vi "Image Label.vi"() -> ()   [LabVIEW 2016]
doc: "This example shows how to label a binary image that contains multiple particles. The labeling process assigns a unique value to all the pixels that belong to a particle. Some processing functions in NI Vision require the input binary image to be labeled."
uses:
  <vilib>/vision/NI_Vision_Development_Module.lvlib
panel:
  out "Number of Particles Found":i32
  out "Extracted Image":T1(plugin-control) caption="Extracted Image (displayed using binary palette)"
  out "Image Source":T1(plugin-control)
  in  "Threshold Values":T2={"Minimum Value"=0.0, "Maximum Value"=150.0}
  in  "Connectivity":bool
  # "Overview: Demonstrates how to threshold an image, smooth the contours of the particles found using an Auto-Median morphological operator, and label the image.\nRequirements: NI Vision Development Module\nInstructions: Run the VI."
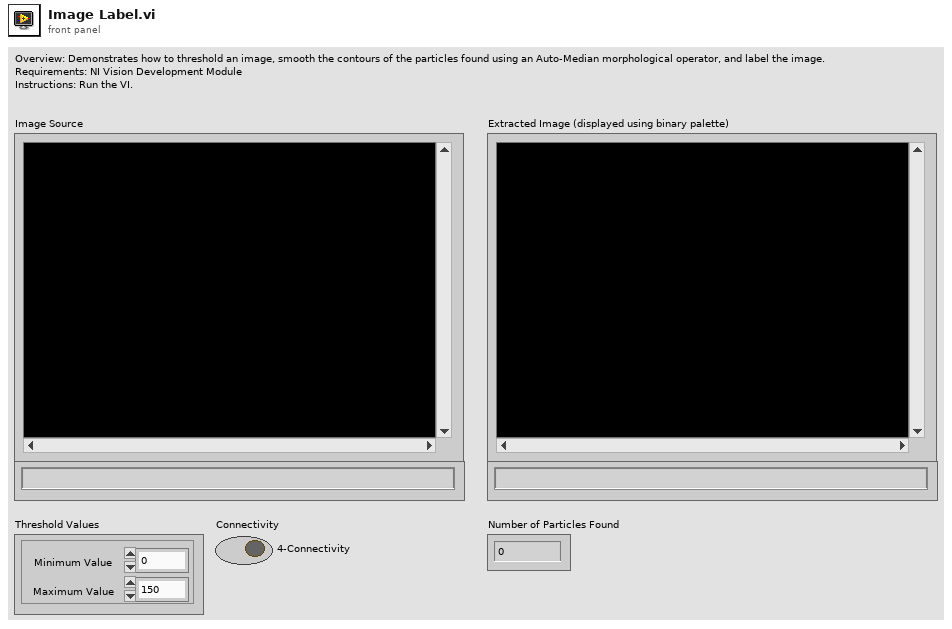
[diagram p1: front panel]
types:
  T1 = typedef "IMAQ Image.ctl" = refnum<image>
  T2 = cluster{"Minimum Value":sgl, "Maximum Value":sgl}
  T3 = enum32{"AutoM", "Close", "Dilate", "Erode", "Gradient", "Gradient out", "Gradient in", "Hit miss", "Open", "PClose", "POpen", "Thick", "Thin"}
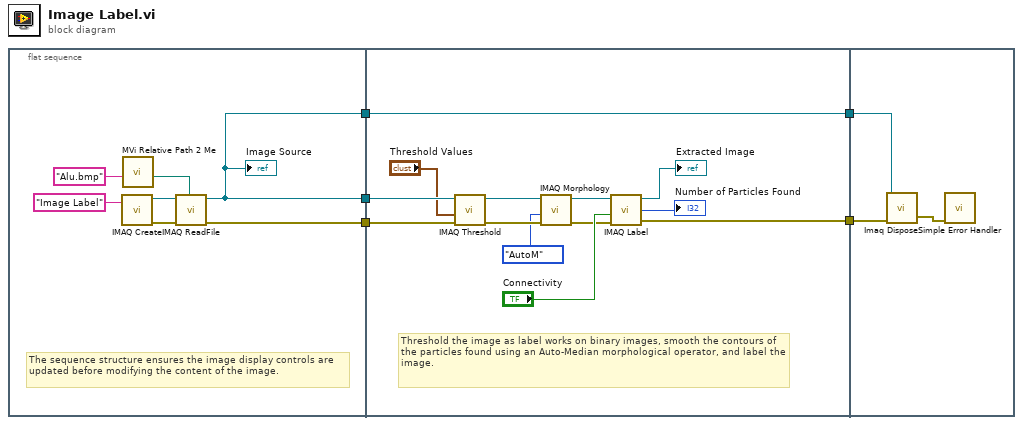
[diagram p0: block diagram]
diagram:
  n1 = flat-sequence {
    tunnel: [w9] -> w4
    tunnel: [w8] -> w3
    tunnel: [w8] -> w1
    tunnel: [w19] -> w5
    tunnel: w4 -> [w18]
    tunnel: w3 -> [w17]
    tunnel: [w16] -> w2
    tunnel: w1 -> [w16]
    tunnel: w5 -> [w28]
    tunnel: w2 -> [w26]
    frame #0 {
      # "The sequence structure ensures the image display controls are updated before modifying the content of the image."
      n2 = call "IMAQ Create"("Image Name"="Image Label") -> ("New Image"=w10:T1, "error out"=w11:errorcluster)  [unwired: 4 in]
      n3 = call "MVi Relative Path 2 Me.vi"("Relative Path"="Alu.bmp" ("name or relative path")) -> ("Appended Dir"=w6:path)  [unwired: 5 in, 1 out]
      n4 = call "IMAQ ReadFile"("File Path"=w6, "error in (no error)"=w11, "Image"=w10) -> ("error out"=w9:errorcluster, "Image Out"=w8:T1)  [unwired: 4 in, 3 out]
      "Image Source" <- w8
    }
    frame #1 {
      # "Threshold the image as label works on binary images, smooth the contours of the particles found using an Auto-Median morphological operator, and label the image."
      n5 = call "IMAQ Threshold"("error in (no error)"=w18, "Range"="Threshold Values", "Image Src"=w17) -> ("error out"=w22:errorcluster, "Image Dst Out"=w25:T1)  [unwired: 7 in]
      n6 = call "IMAQ Morphology"("error in (no error)"=w22, "Operation"=T3."AutoM", "Image Src"=w25) -> ("error out"=w21:errorcluster, "Image Dst Out"=w23:T1)  [unwired: 7 in]
      n7 = call "IMAQ Label"("error in (no error)"=w21, "Connectivity 4/8 (8)"="Connectivity", "Image Src"=w23) -> ("error out"=w19:errorcluster, "Number of Particles"=→"Number of Particles Found":i32, "Image Dst Out"=→"Extracted Image":T1)  [unwired: 1 in]
    }
    frame #2 {
      n8 = call "Imaq Dispose"("Image"=w26, "error in (no error)"=w28) -> ("error out"=w27:errorcluster)  [unwired: 4 in]
      n9 = call <vilib>:"Simple Error Handler.vi"("error in (no error)"=w27) -> ()  [unwired: 4 in, 5 out]
    }
  }
